vi "Main.vi"   [LabVIEW 2020, in "Main.lvclass"]
uses:
  Main.lvclass
  Main.lvclass/Main.ctl
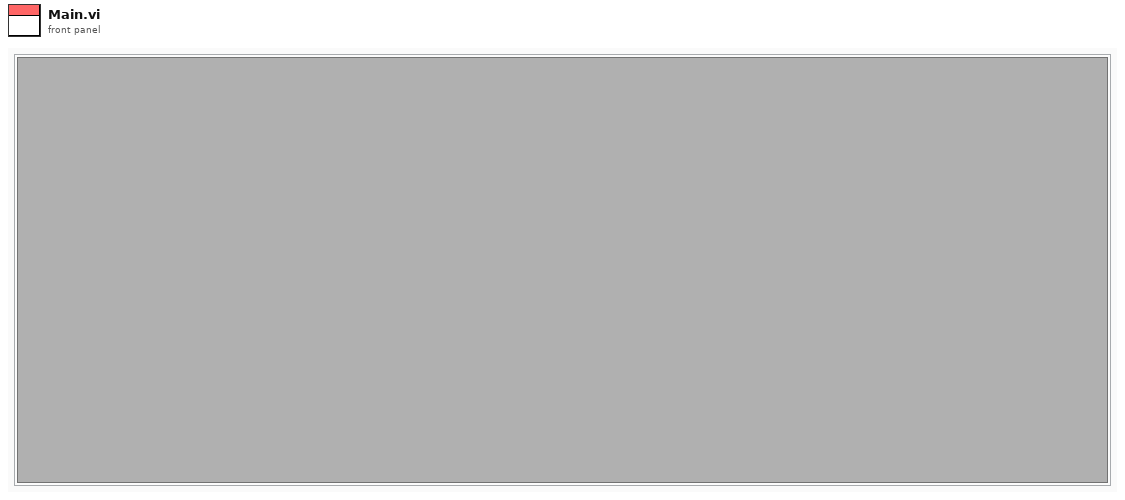
[diagram p1: front panel]
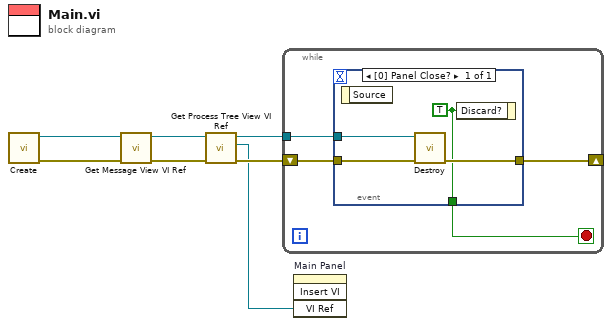
[diagram p0: block diagram]
diagram:
  n1 = call "Create.vi"() -> ("error out"=w7:errorcluster, "Main out"=w5:refnum<class "Main.lvclass">)  [unwired: 10 in]
  n2 = call "Get Message View VI Ref.vi"("error in (no error)"=w7, "Main In"=w5) -> ("error out"=w6:errorcluster, "Main Out"=w2:refnum<class "Main.lvclass">)  [unwired: 7 in, 1 out]
  n3 = call "Get Process Tree View VI Ref.vi"("error in (no error)"=w6, "Main In"=w2) -> ("error out"=w4:errorcluster, "VI Ref"=w1:refnum<vi>, "Main Out"=w3:refnum<class "Main.lvclass">)  [unwired: 7 in]
  n4 = while {
    tunnel: w3 -> [w9]
    shift-right: [w11] -> _
    shift-left: w4 -> [w10]
    stop <- w8 stop-if-true
    n5 = event shown="[0] Panel Close?" {
      selector: _ -> [_]
      dyn-events: _ -> [_]
      timeout: _ -> [_]
      tunnel: [w15] -> w11
      tunnel: w10 -> [w14]
      tunnel: w9 -> [w13]
      tunnel: [w12] -> w8
      event Panel Close? {
        w12 = TRUE ("Discard?")
        n6 = event-data() -> ()  [unwired: 1 in, 1 out]
        n7 = call "Destroy.vi"("error in (no error)"=w14, "Main in"=w13) -> ("error out"=w15:errorcluster)  [unwired: 9 in]
        n8 = event-data("Discard?"=w12) -> ()  [unwired: 1 in, 1 out]
      }
    }
  }
  n9 = invoke on="Main Panel" class="SubPnl" method="Insert VI"("VI Ref"=w1) -> ()  [unwired: 3 in, 4 out]
